vi "Translator.File.Read.FP.vi"(4 "progressbar2":refnum<vi>, 5 "init":bool, 6 "progressbar1":refnum<vi>, 7 "Message":refnum<vi>, 8 "error in":errorcluster, 9 "font name":string, 11 "Translation file":path=path "D:/PL_0125_Sapphire_Automation_branches/SOFTWARE_v1.1-Translation/settings/Translation-Chinese.ini") -> (0 "error out":errorcluster)   [LabVIEW 2016]
uses:
  Translator.Message.ctl
  Translator.Control.Fglb.Action.vi
  Translator.Global.vi
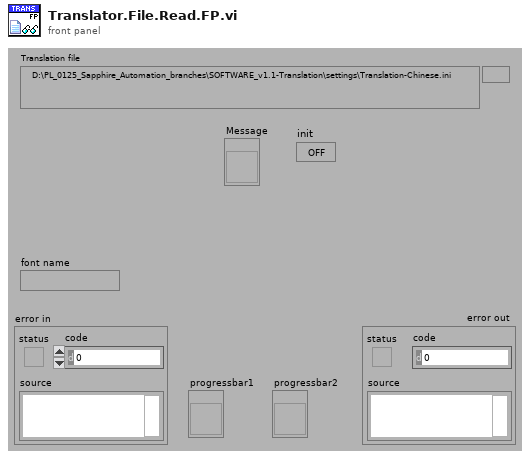
[diagram p1: front panel]
types:
  T1 = typedef "Translator.Message.ctl" = enum16{"-", "Event confirmed", "Log out", "Log in", "Shutdown", "Cancel", "Start", "Continue", "Stop", "On", "Off", "OK", "NOK", "NOK %s", "This", "Prev", "Home", "Work", "In progress...", "Missing", "Empty", "Hardware failure", "Initial", "Error %d >> %s", "Error %d >> %s >> %s", "Starting %s", "Quitting %s", "Configured", "Initializing", "Quitting", "Loading", "Running %s", "Stopped", "Summary", "Do you want to continue?", "Do you want to exit?", "Log out?", "System", "All", "IDLE", "Translating...%s", "Not found", "Alarm %s", "Run", "Skip", "Abort", "Repeat", "Please wait...", "Database disconnected", "Login to database successful", "Login to database failed: %d; %s", "Get process step data for %s", "Changeover off", "Changeover into %s", "Product %s | %s found in cache with status %d at previous station", "Product %s | %s found in database with status %d at previous station", "Product %s | %s not found in cache at previous station", "Product %s | %s not found in database at previous station", "Product %s | %s found in cache with status %d at this station (%d repetion)", "Product %s | %s found in database with status %d at this station (%d repetition)", "Product %s | %s not found in cache at this station", "Product %s | %s not found in database at this station", "Product %s | %s found in cache for component %s | %s", "Product %s | %s found in database for component %s | %s", "Product not found in cache for component %s | %s", "Product not found in database for component %s | %s", "Product %s | %s connected with component %s | %s (cache)", "Product %s | %s connected with component %s | %s (database)", "New data for %s | %s (cache)", "New data for %s | %s (database)", "File %s moved (cache)", "File %s deleted (cache)", "Msg %d >> %s", "PLC LifeBit Failure", "Reconnecting DB", "Reconnecting PLC", "Free disk space is below 1GB - contact technician"}
  T2 = typedef "Translator.Control.Fglb.Action.vi" = enum16{"init", "set", "get", "clear"}
  T3 = typedef "Translator.ControlData.ctl" = cluster{"ref":refnum<vi>, "strict?":bool, "save font?":bool, "type":T4, "root":string, "label":string, "caption":string, "bln.false":string, "bln.true":string, "cols":string[], "rows":string[]}
  T4 = typedef "Translator.ControlTypes.ctl" = enum16{"Cluster", "Array", "Boolean", "Ring", "String", "Tab", "Listbox", "Multicolumn listbox", "Table", "Tree", "Other"}
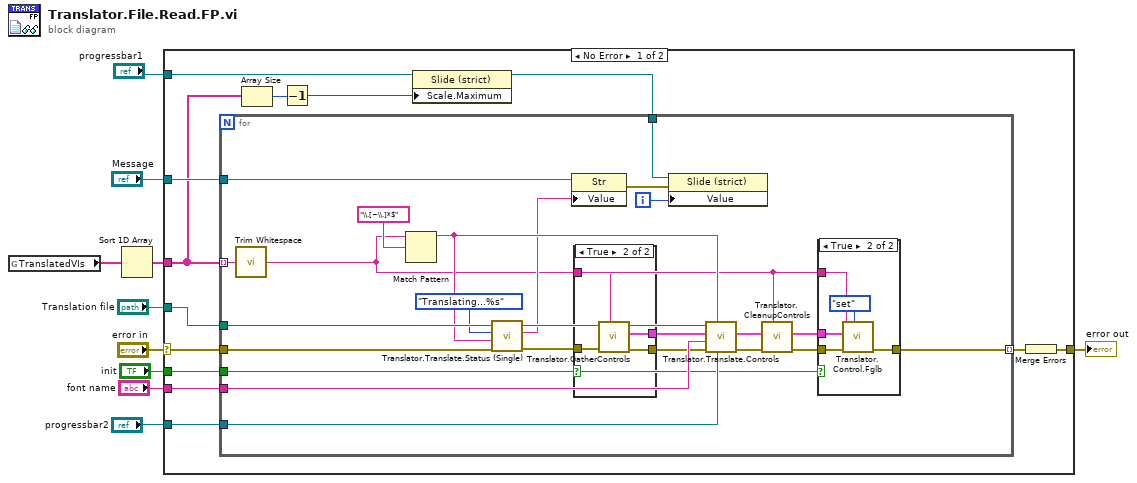
[diagram p0: block diagram]
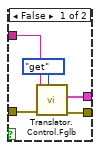
[diagram p3: hidden frame]
diagram:
  n1 = global read "Translator.Global.vi" "TranslatedVIs"() -> (w2:string[])
  n2 = Sort 1D Array(array=w2) -> (sorted array=w3:string[])
  n3 = case shown="No Error" "error in" {
    selector: "error in" -> [w22 w60]
    tunnel: "Translation file" -> [w20 _]
    tunnel: [w12 w60] -> w9
    tunnel: w3 -> [w15 _]
    tunnel: "font name" -> [w23 _]
    tunnel: "progressbar2" -> [w19 _]
    tunnel: "Message" -> [w18 _]
    tunnel: "progressbar1" -> [w14 _]
    tunnel: "init" -> [w11 _]
    frame No Error {
      n4 = Array Size(array=w15) -> (size(s)=w17:i32)
      n5 = Decrement(x=w17) -> (x-1=w16:i32)
      n6 = property on="Property Node" class="Slide (strict)"(reference=w14, "Scale.Maximum"=w16) -> (reference out=w13:refnum<vi>)  [unwired: 1 in, 1 out]
      n7 = for {
        tunnel: w15 -> [w43] mode=indexing
        tunnel: w23 -> [w44]
        tunnel: w20 -> [w38]
        tunnel: w19 -> [w42]
        tunnel: w18 -> [w41]
        tunnel: w13 -> [w40]
        tunnel: w22 -> [w25]
        tunnel: [w24] -> w21 mode=indexing
        tunnel: w11 -> [w37]
        i -> [w39]
        n8 = call <vilib>:"Trim Whitespace.vi"("string"=w43) -> ("trimmed string"=w26:string)  [unwired: 1 in]
        n9 = Match Pattern(string=w26, regular expression="\\.[~\\.]*$") -> (before substring=w30:string)  [unwired: 4 out]
        n10 = call "Translator.Translate.Status (Single).vi"("error in (no error)"=w25, "Arg"=w30, "Msg"=Translator.Message."Translating...%s" ("msg")) -> ("error out"=w33:errorcluster, "Translated Msg"=w29:string)  [unwired: 7 in]
        n11 = property class="Str"(reference=w41, "Value"=w29) -> (error out=w34:errorcluster)  [unwired: 1 in, 1 out]
        n12 = case shown="True" w37 {
          tunnel: [w54 w59] -> w36
          tunnel: w33 -> [w53 w58]
          tunnel: [w52 w57] -> w28
          tunnel: w26 -> [w51 w56]
          frame False {
            n13 = call "Translator.Control.Fglb.vi"("Action"=Translator.Control.Fglb.Action.vi."get", "error in (no error)"=w53, "VI name"=w51) -> ("error out"=w54:errorcluster, "Controls out"=w52:T3[])  [unwired: 7 in]
          }
          frame True {
            n14 = call "Translator.GatherControls.vi"("VI name"=w56, "error in"=w58) -> ("error out"=w59:errorcluster, "Controls out"=w57:T3[])  [unwired: 8 in]
          }
        }
        n15 = property on="Property Node" class="Slide (strict)"(reference=w40, error in=w34, "Value"=w39) -> ()  [unwired: 2 out]
        n16 = call "Translator.Translate.Controls.vi"("progressbar"=w42, "group"=w30, "error in"=w36, "font name"=w44, "Controls out"=w28, "Translation file"=w38) -> ("error out"=w35:errorcluster)  [unwired: 5 in]
        n17 = call "Translator.CleanupControls.vi"("VI name"=w26, "error in"=w35, "Controls"=w28) -> ("error out"=w27:errorcluster)  [unwired: 8 in]
        n18 = case shown="True" w37 {
          tunnel: w28 -> [_ w50]
          tunnel: w26 -> [_ w49]
          tunnel: w27 -> [w45 w47]
          tunnel: [w45 w46] -> w24
          frame False {
          }
          frame True {
            n19 = call "Translator.Control.Fglb.vi"("Action"=Translator.Control.Fglb.Action.vi."set", "error in (no error)"=w47, "Controls in"=w50, "VI name"=w49) -> ("error out"=w46:errorcluster)  [unwired: 6 in, 1 out]
          }
        }
      }
      n20 = Merge Errors(w21) -> (w12:errorcluster)
    }
    frame Error {
    }
  }
  "error out" <- w9
